vi "Test Error Logger.vi"(8 "error in (no error)":errorcluster) -> (0 "error out":errorcluster)   [LabVIEW 2019]
uses:
  <userlib>/LevyLab/Logger.Error/Logger.Error.lvclass
  <vilib>/addons/_JKI Toolkits/Caraya/classes/Assert/Assert Not Error.vi
  <vilib>/Utility/file.llb/Write Delimited Spreadsheet (string).vi
  <vilib>/Utility/file.llb/Read Delimited Spreadsheet (string).vi
  <vilib>/addons/_JKI Toolkits/Caraya/classes/Assert/Assert Equal Value and Type_Variant.vi
  <vilib>/addons/_JKI Toolkits/Caraya/classes/Assert/Assert.lvclass
  <vilib>/addons/_JKI Toolkits/Caraya/classes/Test/Test.lvclass
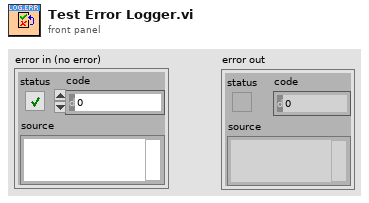
[diagram p1: front panel]
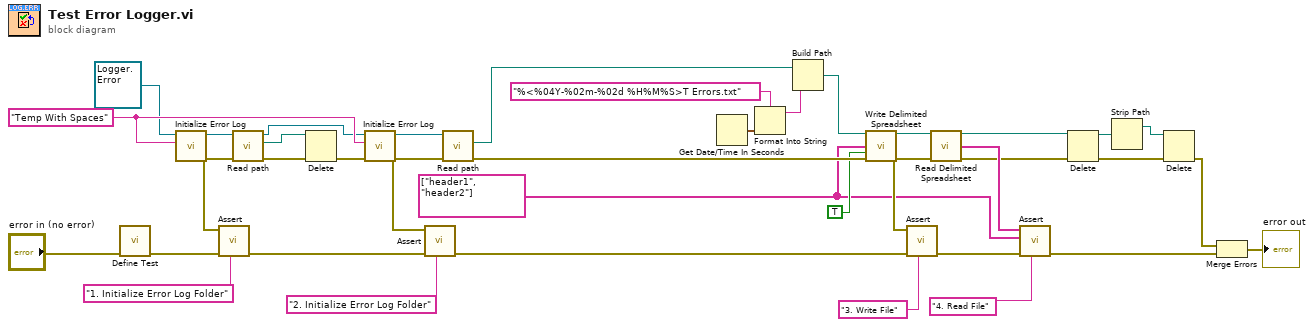
[diagram p0: block diagram]
diagram:
  w3 = string[] ["header1", "header2"] ("1D data")
  w31 = "Temp With Spaces" ("name or relative path")
  n1 = call <vilib>:"Define Test.vi"("error in (no error)"="error in (no error)") -> ("error out"=w35:errorcluster)  [unwired: 9 in, 1 out]
  n2 = call <userlib>:"Initialize Error Log.vi"("Application Name"=w31, "Logger.Error in"=refnum<class "Logger.Error.lvclass"> refnum) -> ("error out"=w30:errorcluster, "Logger.Error out"=w37:refnum<class "Logger.Error.lvclass">)  [unwired: 8 in]
  n3 = call-poly <vilib>:"Assert.vi"("Label"="1. Initialize Error Log Folder", "error in (no error)"=w35, "Not Error?"=w30) -> ("error out"=w29:errorcluster)  [unwired: 7 in, 1 out]
  n4 = call-dynamic "Read path.vi"("error in (no error)"=w30, "Logger in"=w37) -> ("error out"=w33:errorcluster, "path"=w34:path, "Logger out"=w27:refnum<class "Logger.Error.lvclass">)  [unwired: 7 in]
  n5 = Delete(path (use dialog)=w34, error in=w33) -> (error out=w32:errorcluster)  [unwired: 3 in, 2 out]
  n6 = call <userlib>:"Initialize Error Log.vi"("error in (no error)"=w32, "Application Name"=w31, "Logger.Error in"=w27) -> ("error out"=w24:errorcluster, "Logger.Error out"=w25:refnum<class "Logger.Error.lvclass">)  [unwired: 7 in]
  n7 = call-poly <vilib>:"Assert.vi"("Label"="2. Initialize Error Log Folder", "error in (no error)"=w29, "Not Error?"=w24) -> ("error out"=w21:errorcluster)  [unwired: 7 in, 1 out]
  n8 = call-dynamic "Read path.vi"("error in (no error)"=w24, "Logger in"=w25) -> ("error out"=w23:errorcluster, "path"=w5:path)  [unwired: 7 in, 1 out]
  n9 = Get Date/Time In Seconds() -> (seconds since 1Jan1904=w4:timestamp)
  n10 = Format Into String(format string="%<%04Y-%02m-%02d %H%M%S>T Errors.txt", w4) -> (resulting string=w6:string)  [unwired: 2 in, 1 out]
  n11 = Build Path(base path=w5, name or relative path=w6) -> (appended path=w2:path)
  n12 = call-poly <vilib>:"Write Delimited Spreadsheet.vi"("file path (dialog if empty)"=w2, "1D data"=w3, "append to file? (new file:F)"=TRUE, "error in (no error)"=w23) -> ("new file path (Not A Path if cancelled)"=w19:path, "error out"=w20:errorcluster)  [unwired: 10 in]
  n13 = call-poly <vilib>:"Assert.vi"("Label"="3. Write File", "error in (no error)"=w21, "Not Error?"=w20) -> ("error out"=w16:errorcluster)  [unwired: 7 in, 1 out]
  n14 = call-poly <vilib>:"Read Delimited Spreadsheet.vi"("file path (dialog if empty)"=w19, "error in (no error)"=w20) -> ("new file path (Not A Path if cancelled)"=w14:path, "first row"=w17:string[], "error out"=w1:errorcluster)  [unwired: 8 in, 3 out]
  n15 = call-poly <vilib>:"Assert.vi"("Label"="4. Read File", "error in (no error)"=w16, "Y"=w3, "X"=w17) -> ("error out"=w12:errorcluster)  [unwired: 6 in, 1 out]
  n16 = Delete(path (use dialog)=w14, error in=w1) -> (deleted path=w11:path, error out=w9:errorcluster)  [unwired: 3 in, 1 out]
  n17 = Strip Path(path=w11) -> (stripped path=w10:path)  [unwired: 1 out]
  n18 = Delete(path (use dialog)=w10, error in=w9) -> (error out=w8:errorcluster)  [unwired: 3 in, 2 out]
  n19 = Merge Errors(w8, w12) -> (→"error out":errorcluster)
